vi "Pockels Cal-Cal range entry initialisation.vi"(11 "Cluster":T1) -> (0 "error out":errorcluster, 3 "XYGraph out":refnum<vi>)   [LabVIEW 2017]
uses:
  Globals/gl_Calibration globals.vi
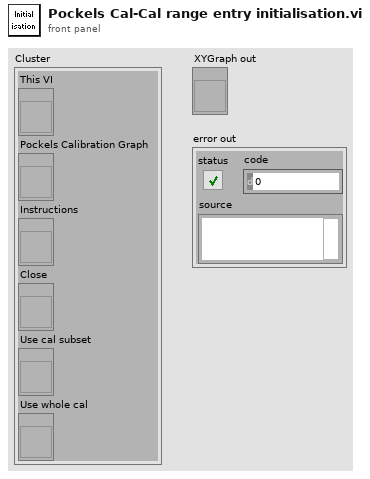
[diagram p1: front panel]
types:
  T1 = cluster{"This VI":refnum<vi>, "Pockels Calibration Graph":refnum<vi>, "Instructions":refnum<vi>, "Close":refnum<vi>, "Use cal subset":refnum<vi>, "Use whole cal":refnum<vi>}
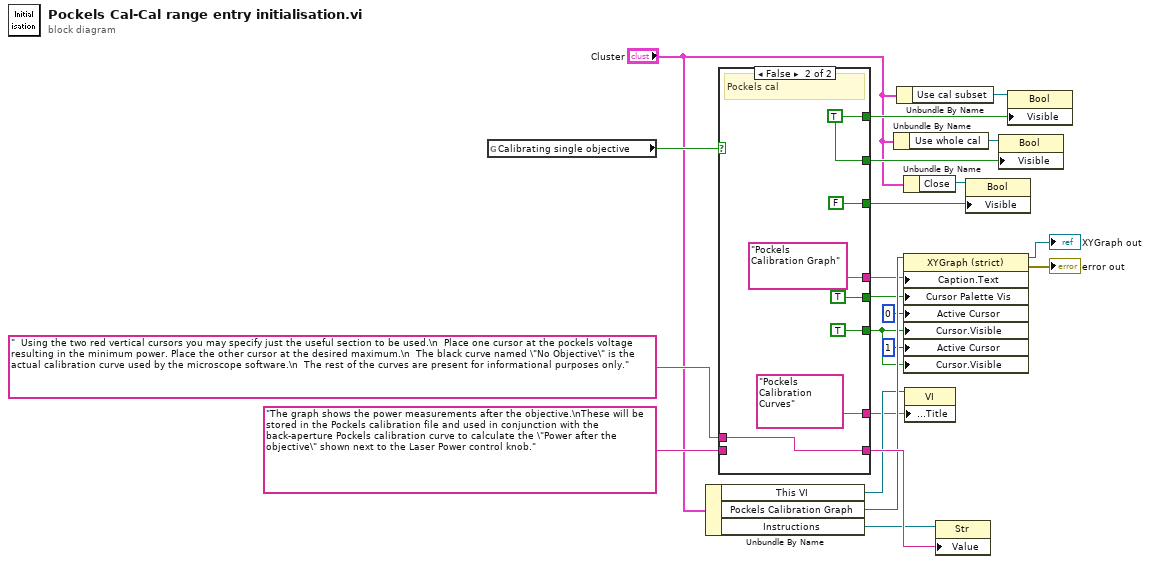
[diagram p0: block diagram]
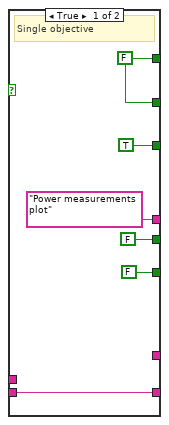
[diagram p2: hidden frame]
diagram:
  n1 = global read "gl_Calibration globals.vi" "Calibrating single objective"() -> (w2:bool)
  n2 = Unbundle By Name("Cluster") -> ("This VI"=w15:refnum<vi>, "Pockels Calibration Graph"=w16:refnum<vi>, "Instructions"=w17:refnum<vi>)
  n3 = case shown="False" w2 {
    tunnel: [TRUE FALSE] -> w3
    tunnel: [w27 w34] -> w4
    tunnel: [w27 w34] -> w5
    tunnel: [w26 w33] -> w18
    tunnel: "  Using the two red vertical cursors you may specify just the useful section to be used.\n  Place one cursor at the pockels voltage resulting in the minimum power. Place the other cursor at the desired maximum.\n  The black curve named \"No Objective\" is the actual calibration curve used by the microscope software.\n  The rest of the curves are present for informational purposes only." ("Instructions") -> [_ w33]
    tunnel: "The graph shows the power measurements after the objective.\nThese will be stored in the Pockels calibration file and used in conjunction with the back-aperture Pockels calibration curve to calculate the \"Power after the objective\" shown next to the Laser Power control knob." ("Instructions") -> [w26 _]
    tunnel: ["Power measurements plot" ("Label.Text") "Pockels Calibration Graph" ("Label.Text")] -> w9
    tunnel: [FALSE TRUE] -> w8
    tunnel: [_ "Pockels Calibration Curves" ("Front Panel Window:Title")] -> w10
    tunnel: [FALSE TRUE] -> w12
    frame True {
      w27 = FALSE
      # "Single objective"
    }
    frame False {
      w34 = TRUE
      # "Pockels cal"
    }
  }
  n4 = Unbundle By Name("Cluster") -> ("Use whole cal"=w22:refnum<vi>)
  n5 = Unbundle By Name("Cluster") -> ("Use cal subset"=w21:refnum<vi>)
  n6 = Unbundle By Name("Cluster") -> ("Close"=w20:refnum<vi>)
  n7 = property on="Property Node" class="XYGraph (strict)"(reference=w16, "Caption.Text"=w9, "Cursor Palette Vis"=w8, "Active Cursor"=u32 0, "Cursor.Visible"=w12, "Active Cursor"=u32 1, "Cursor.Visible"=w12) -> (reference out=→"XYGraph out":refnum<vi>, error out=→"error out":errorcluster)  [unwired: 1 in]
  n8 = property on="Property Node" class="VI"(reference=w15, "Front Panel.Title"=w10) -> ()  [unwired: 1 in, 2 out]
  n9 = property on="Property Node" class="Str"(reference=w17, "Value"=w18) -> ()  [unwired: 1 in, 2 out]
  n10 = property on="Property Node" class="Bool"(reference=w20, "Visible"=w3) -> ()  [unwired: 1 in, 2 out]
  n11 = property on="Property Node" class="Bool"(reference=w22, "Visible"=w5) -> ()  [unwired: 1 in, 2 out]
  n12 = property on="Property Node" class="Bool"(reference=w21, "Visible"=w4) -> ()  [unwired: 1 in, 2 out]
